vi "Sequence-Abort.vi"(8 "error in (no error)":errorcluster) -> (0 "error out":errorcluster)   [LabVIEW 2016]
uses:
  Sequence.Action.ctl
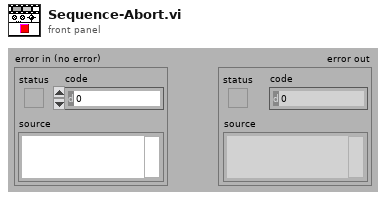
[diagram p1: front panel]
types:
  T1 = typedef "Sequence.Action.ctl" = enum32{"idle", "constructor", "destructor", "--- Sequence ---", "Abort", "Init", "Select", "Start", "Work.Run", "Work.AirON", "Work.LaserON", "Work.Done", "Process.Run", "Process.Engine", "Process.Pause", "Process.DoorLock", "Process.Wait4Container", "Process.Wait1", "Process.Wait2", "Process.Continue", "Process.Done", "Home.Run", "Home.AirON", "Home.TablePos", "Home.MoveServo", "Home.LaserOFF", "Home.AirOFF", "Home.Done", "User.Action", "User.Data", "Status.Clear"}
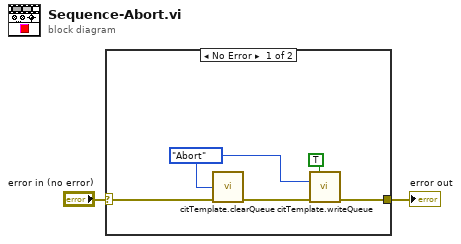
[diagram p0: block diagram]
diagram:
  n1 = case shown="No Error" "error in (no error)" {
    selector: "error in (no error)" -> [w5 w8]
    tunnel: [w7 w8] -> w1
    frame No Error {
      w3 = Sequence.Action."Abort" ("Action")
      n2 = call "citTemplate.clearQueue.vi"("event in"=w3, "error in (no error)"=w5) -> ("error out"=w4:errorcluster)  [unwired: 12 in, 1 out]
      n3 = call "citTemplate.writeQueue.vi"("High priority (F)"=TRUE, "event in (if not connected:all statemachine with data event)"=w3, "error in (no error)"=w4) -> ("error out"=w7:errorcluster)  [unwired: 12 in]
    }
    frame Error {
    }
  }
  "error out" <- w1
